vi "Print.vi"(8 "error in (no error)":errorcluster, 11 "Message Double in":refnum<class "Message Double and Boolean Array.lvclass">) -> (0 "error out":errorcluster, 2 "String":string, 3 "Message Double out":refnum<class "Message Double and Boolean Array.lvclass">)   [LabVIEW 2016, in "WebSocket Networking.lvlib" / "Message Double and Boolean Array.lvclass"]
doc: "--\nCopyright © 2017 Composed SystemsI All rights reserved.\n\nAuthor: Jon McBee <jon.mcbee@composed.io>\n\nThis library is provided \"AS IS\" ,WITHOUT WARRANTIES OR\nCONDITIONS OF ANY KIND, either express or implied.\n\nComposed Systems -- composed.io\n\nStream 0.0.1.1\nJon McBee - Composed Systems\nCopyright (c) 2017, Composed Systems"
uses:
  <userlib>/Common Components/WebSocket Networking/Message Double and Boolean Array/Message Double and Boolean Array.lvclass
  C:/Program Files (x86)/National Instruments/LabVIEW 2016/user.lib/Composed Systems/Stream/Mediator/Classes/Message Interface/Message Interface.lvclass
  <userlib>/Common Components/WebSocket Networking/Message Double and Boolean Array/Message Double and Boolean Array.lvclass/Message Double and Boolean Array.ctl
  <userlib>/Composed Systems/Stream/Mediator/Classes/Message Interface/Message Interface.lvclass
  <vilib>/addons/_JKI.lib/Serialization/JSON/JKI JSON Serialization.lvlib
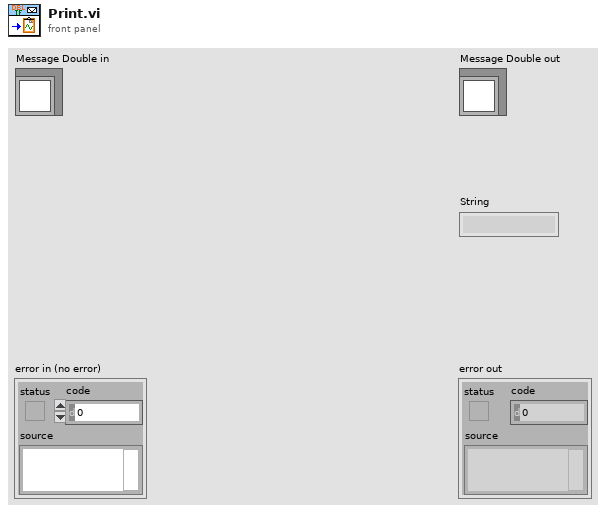
[diagram p1: front panel]
types:
  T1 = typedef "WebSocket Networking.lvlib/Message Double and Boolean Array.lvclass/Value.ctl" = cluster{"Master ID":string, "Doubles":dbl[], "Booleans":bool[]}
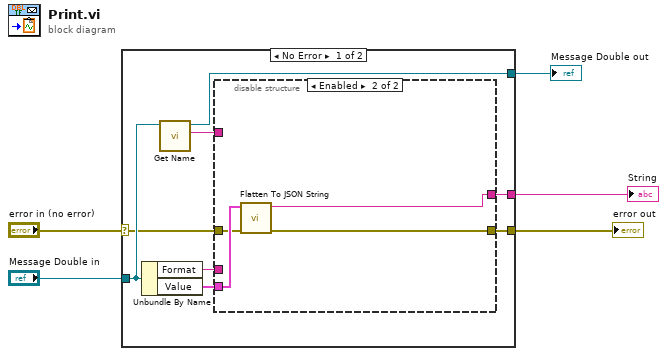
[diagram p0: block diagram]
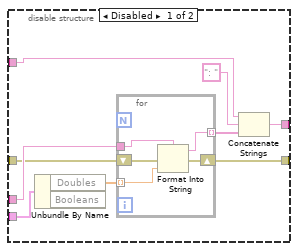
[diagram p2: hidden frame]
diagram:
  n1 = case shown="No Error" "error in (no error)" {
    selector: "error in (no error)" -> [w9 w32]
    tunnel: [w8 w32] -> w4
    tunnel: [w12 w33] -> w2
    tunnel: "Message Double in" -> [w13 w33]
    tunnel: [w6 _] -> w1
    frame No Error {
      n2 = Unbundle By Name(w13) -> ("Format"=w11:string, "Value"=w10:T1)
      n3 = call <userlib>:"Get Name.vi"("Message Interface in"=w13) -> ("Name"=w7:string, "Message Interface out"=w12:refnum<class "Message Double and Boolean Array.lvclass">)  [unwired: 8 in, 1 out]
      n4 = disable-structure shown="Enabled" {
        disable-tunnel: w11 -> [w22 _]
        disable-tunnel: w10 -> [w21 w31]
        disable-tunnel: w9 -> [w20 w30]
        disable-tunnel: [w19 w29] -> w8
        disable-tunnel: w7 -> [w18 _]
        disable-tunnel: [w15 w28] -> w6
        frame Disabled {
          n5 = Unbundle By Name(w21) -> ("Doubles"=w14:dbl[])  [unwired: 1 out]
          n6 = for {
            tunnel: w22 -> [w27]
            tunnel: w14 -> [w26] mode=indexing
            shift-right: [w24] -> w19
            shift-left: w20 -> [w25]
            tunnel: [w23] -> w16 mode=indexing
            n7 = Format Into String(format string=w27, error in=w25, w26) -> (resulting string=w23:string, error out=w24:errorcluster)  [unwired: 1 in]
          }
          n8 = Concatenate Strings(w18, ": ", w16) -> (w15:string)
        }
        frame Enabled {
          n9 = call <vilib>:"Flatten To JSON String.vi"("error in (no error)"=w30, "Variant"=w31) -> ("error out"=w29:errorcluster, "JSON String"=w28:string)  [unwired: 8 in]
        }
      }
    }
    frame Error {
    }
  }
  "error out" <- w4
  "Message Double out" <- w2
  "String" <- w1
